vi "Sub.vi"(8 "error in (no error)":errorcluster caption="错误输入（无错误）", 10 "Size 输入":refnum<class "Size.lvclass"> caption="DNL_LabVIEW Object in", 11 "Size 输入":refnum<class "Size.lvclass"> caption="DNL_LabVIEW Object in") -> (0 "error out":errorcluster caption="错误输出", 3 "Size 输出":refnum<class "Size.lvclass"> caption="DNL_LabVIEW Object out")   [LabVIEW 2011, in "Size.lvclass"]
uses:
  Size.lvclass
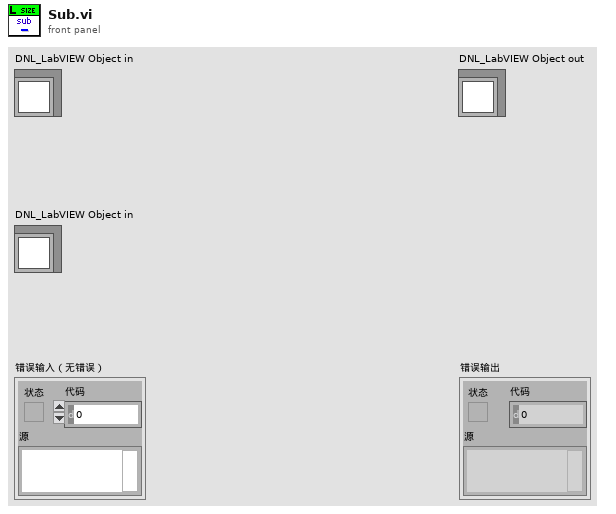
[diagram p1: front panel]
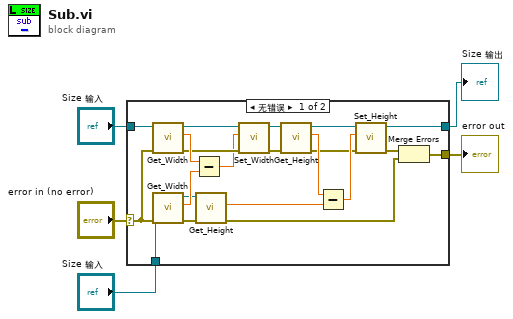
[diagram p0: block diagram]
diagram:
  n1 = case shown="无错误" "error in (no error)" {
    selector: "error in (no error)" -> [w9 w28]
    tunnel: [w6 w28] -> w4
    tunnel: [w10 w27] -> w2
    tunnel: "Size 输入" -> [w26 w27]
    tunnel: "Size 输入" -> [w25 _]
    frame No Error {
      n2 = call "Get_Width.vi"("error in (no error)"=w9, "Size输入"=w26) -> ("error out"=w21:errorcluster, "Width"=w24:dbl, "Size输出"=w22:refnum<class "Size.lvclass">)  [unwired: 7 in]
      n3 = call "Get_Width.vi"("error in (no error)"=w9, "Size输入"=w25) -> ("error out"=w18:errorcluster, "Width"=w23:dbl, "Size输出"=w19:refnum<class "Size.lvclass">)  [unwired: 7 in]
      n4 = Subtract(x=w24, y=w23) -> (x-y=w20:dbl)
      n5 = call "Get_Height.vi"("error in (no error)"=w18, "Size输入"=w19) -> ("error out"=w7:errorcluster, "Height"=w14:dbl)  [unwired: 7 in, 1 out]
      n6 = call "Set_Width.vi"("error in (no error)"=w21, "Width"=w20, "Size输入"=w22) -> ("error out"=w16:errorcluster, "Size输出"=w17:refnum<class "Size.lvclass">)  [unwired: 7 in]
      n7 = call "Get_Height.vi"("error in (no error)"=w16, "Size输入"=w17) -> ("error out"=w11:errorcluster, "Height"=w15:dbl, "Size输出"=w13:refnum<class "Size.lvclass">)  [unwired: 7 in]
      n8 = Subtract(x=w15, y=w14) -> (x-y=w12:dbl)
      n9 = call "Set_Height.vi"("error in (no error)"=w11, "Height"=w12, "Size输入"=w13) -> ("error out"=w8:errorcluster, "Size输出"=w10:refnum<class "Size.lvclass">)  [unwired: 7 in]
      n10 = Merge Errors(w8, w7) -> (w6:errorcluster)
    }
    frame Error {
    }
  }
  "error out" <- w4
  "Size 输出" <- w2
